vi "execute.vi"(8 "error in (no error)":errorcluster, 9 "trajectory in":refnum<class "GenericComponent.lvclass">, 10 "imaging mode in":refnum<class "GenericComponent.lvclass">, 11 "adapter in":refnum<class "AdapterTS090826ImagingModeToTrajectory.lvclass">) -> (0 "error out":errorcluster, 1 "trajectory out":refnum<class "GenericComponent.lvclass">, 2 "imaging mode out":refnum<class "GenericComponent.lvclass">, 3 "adapter out":refnum<class "AdapterTS090826ImagingModeToTrajectory.lvclass">)   [LabVIEW 2010, in "AdapterTS090826ImagingModeToTrajectory.lvclass"]
uses:
  AdapterTS090826ImagingModeToTrajectory.lvclass
  common/classes/GenericComponent/GenericComponent/GenericComponent.lvclass
  ImagingMode/ImagingModeTS090821Circular2D/ImagingModeTS090821Circular2D/ImagingModeTS090821Circular2D.lvclass
  Trajectory/TrajectoryTS090820Circular2D/TrajectoryTS090820Circular2D/TrajectoryTS090820Circular2D.lvclass
panel:
  # "imaging mode: ImagingModeTS090821Circular2D\ntrajectory: TrajectoryTS090820Circular2D"
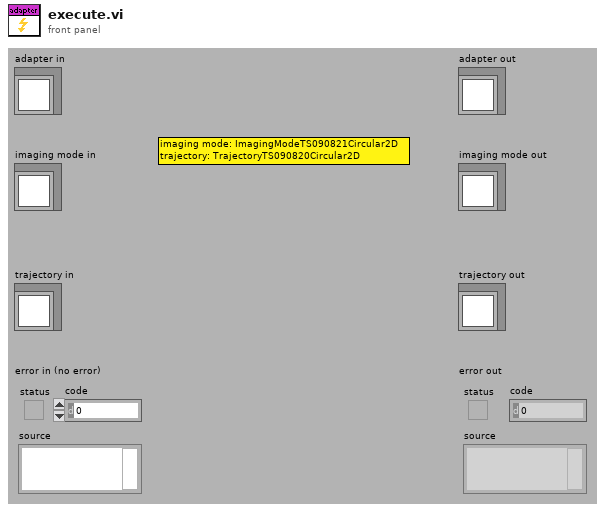
[diagram p1: front panel]
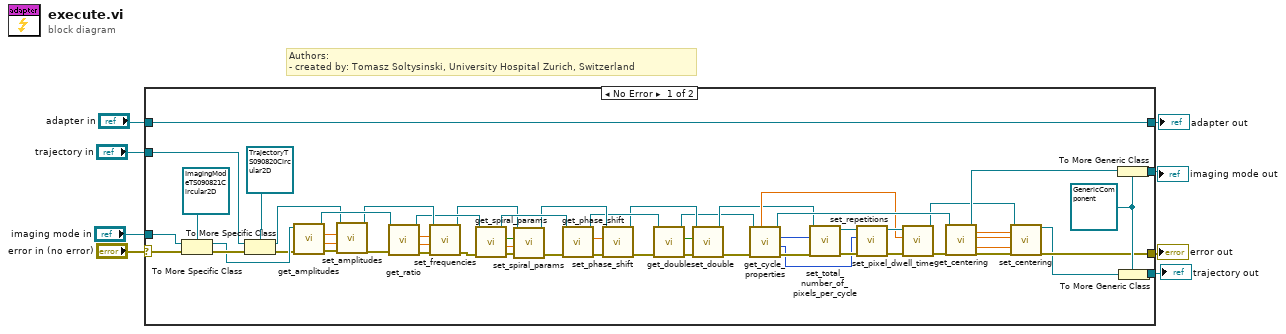
[diagram p0: block diagram]
diagram:
  # "Authors: \n- created by: Tomasz Soltysinski, University Hospital Zurich, Switzerland"
  n1 = case shown="No Error" "error in (no error)" {
    selector: "error in (no error)" -> [w65 w70]
    tunnel: [w67 w71] -> w6
    tunnel: "adapter in" -> [w67 w71]
    tunnel: "imaging mode in" -> [w66 w68]
    tunnel: "trajectory in" -> [w63 w69]
    tunnel: [w53 w68] -> w2
    tunnel: [w33 w70] -> w3
    tunnel: [w54 w69] -> w1
    frame No Error {
      w60 = refnum<class "GenericComponent.lvclass"> refnum ("GenericComponent.lvclass")
      n2 = To More Specific Class(target class=refnum<class "ImagingModeTS090821Circular2D.lvclass"> refnum, reference=w66, error in=w65) -> (specific class reference=w59:refnum<class "ImagingModeTS090821Circular2D.lvclass">, error out=w64:errorcluster)
      n3 = To More Specific Class(target class=refnum<class "TrajectoryTS090820Circular2D.lvclass"> refnum, reference=w63, error in=w64) -> (specific class reference=w42:refnum<class "TrajectoryTS090820Circular2D.lvclass">, error out=w57:errorcluster)
      n4 = call-dynamic "get_amplitudes.vi"("error in (no error)"=w57, "ScanModeTS090821Circular2D in"=w59) -> ("error out"=w49:errorcluster, "y amplitude"=w45:dbl[unit], "x amplitude"=w46:dbl[unit], "ScanModeTS090821Circular2D out"=w58:refnum<class "ImagingModeTS090821Circular2D.lvclass">)  [unwired: 6 in]
      n5 = call-dynamic "set_amplitudes.vi"("error in (no error)"=w49, "y amplitude"=w45, "x amplitude"=w46, "TrajectoryTS090820Circular2D in"=w42) -> ("error out"=w48:errorcluster, "TrajectoryTS090820Circular2D out"=w50:refnum<class "TrajectoryTS090820Circular2D.lvclass">)  [unwired: 6 in]
      n6 = call-dynamic "get_ratio.vi"("error in (no error)"=w48, "ScanModeTS090821Circular2D in"=w58) -> ("error out"=w47:errorcluster, "y frequency"=w43:dbl, "x frequency"=w44:dbl, "ScanModeTS090821Circular2D out"=w19:refnum<class "ImagingModeTS090821Circular2D.lvclass">)  [unwired: 6 in]
      n7 = call-dynamic "set_frequencies.vi"("error in (no error)"=w47, "y frequency"=w43, "x frequency"=w44, "TrajectoryTS090820Circular2D in"=w50) -> ("error out"=w20:errorcluster, "TrajectoryTS090820Circular2D out"=w18:refnum<class "TrajectoryTS090820Circular2D.lvclass">)  [unwired: 6 in]
      n8 = call-dynamic "get_spiral_params.vi"("error in (no error)"=w20, "ScanModeTS090821Circular2D in"=w19) -> ("error out"=w24:errorcluster, "dump factor"=w21:dbl, "Spiral"=w22:bool, "ScanModeTS090821Circular2D out"=w26:refnum<class "ImagingModeTS090821Circular2D.lvclass">)  [unwired: 6 in]
      n9 = call-dynamic "set_spiral_params.vi"("error in (no error)"=w24, "dump factor"=w21, "Spiral"=w22, "TrajectoryTS090820Circular2D in"=w18) -> ("error out"=w23:errorcluster, "TrajectoryTS090820Circular2D out"=w25:refnum<class "TrajectoryTS090820Circular2D.lvclass">)  [unwired: 6 in]
      n10 = call-dynamic "get_phase_shift.vi"("error in (no error)"=w23, "ScanModeTS090821Circular2D in"=w26) -> ("error out"=w56:errorcluster, "phase shift"=w52:dbl, "ScanModeTS090821Circular2D out"=w16:refnum<class "ImagingModeTS090821Circular2D.lvclass">)  [unwired: 7 in]
      n11 = call-dynamic "set_phase_shift.vi"("error in (no error)"=w56, "Phase shift"=w52, "TrajectoryTS090820Circular2D in"=w25) -> ("error out"=w15:errorcluster, "TrajectoryTS090820Circular2D out"=w14:refnum<class "TrajectoryTS090820Circular2D.lvclass">)  [unwired: 7 in]
      n12 = call-dynamic "get_double.vi"("error in (no error)"=w15, "ImagingModeTS090821Circular2D in"=w16) -> ("error out"=w12:errorcluster, "Double"=w10:bool, "ImagingModeTS090821Circular2D out"=w9:refnum<class "ImagingModeTS090821Circular2D.lvclass">)  [unwired: 7 in]
      n13 = call-dynamic "set_double.vi"("error in (no error)"=w12, "double"=w10, "TrajectoryTS090820Circular2D in"=w14) -> ("error out"=w11:errorcluster, "TrajectoryTS090820Circular2D out"=w13:refnum<class "TrajectoryTS090820Circular2D.lvclass">)  [unwired: 7 in]
      n14 = call-dynamic "get_cycle_properties.vi"("error in (no error)"=w11, "ScanModeTS090821Circular2D in"=w9) -> ("error out"=w55:errorcluster, "number of cycles"=w37:i32, "total number of pixels per cycle"=w51:i32, "ScanModeTS090821Circular2D out"=w32:refnum<class "ImagingModeTS090821Circular2D.lvclass">, "pixel dwell time"=w17:dbl[unit])  [unwired: 3 in, 2 out]
      n15 = call-dynamic "set_total_number_of_pixels_per_cycle.vi"("error in (no error)"=w55, "total number of pixels per cycle"=w51, "TrajectoryTS090820Circular2D in"=w13) -> ("error out"=w41:errorcluster, "TrajectoryTS090820Circular2D out"=w40:refnum<class "TrajectoryTS090820Circular2D.lvclass">)  [unwired: 7 in]
      n16 = call-dynamic "set_repetitions.vi"("error in (no error)"=w41, "repetitions"=w37, "GenericTrajectory in"=w40) -> ("error out"=w38:errorcluster, "GenericTrajectory out"=w39:refnum<class "TrajectoryTS090820Circular2D.lvclass">)  [unwired: 7 in]
      n17 = call-dynamic "set_pixel_dwell_time.vi"("error in (no error)"=w38, "pixel dwell time"=w17, "GenericTrajectory.lvclass in"=w39) -> ("error out"=w36:errorcluster, "GenericTrajectory.lvclass out"=w31:refnum<class "TrajectoryTS090820Circular2D.lvclass">)  [unwired: 7 in]
      n18 = call-dynamic "get_centering.vi"("ScanModeTS090821Circular2D in"=w32, "error in (no error)"=w36) -> ("ScanModeTS090821Circular2D out"=w35:refnum<class "ImagingModeTS090821Circular2D.lvclass">, "x center"=w30:dbl, "y center"=w29:dbl, "rotation angle"=w28:dbl, "error out"=w34:errorcluster)  [unwired: 13 in]
      n19 = call-dynamic "set_centering.vi"("TrajectoryTS090820Circular2D in"=w31, "x center"=w30, "y center"=w29, "rotation angle"=w28, "error in (no error)"=w34) -> ("TrajectoryTS090820Circular2D out"=w27:refnum<class "TrajectoryTS090820Circular2D.lvclass">, "error out"=w33:errorcluster)  [unwired: 13 in]
      n20 = To More Generic Class(target class=w60, reference=w35) -> (generic class reference=w53:refnum<class "GenericComponent.lvclass">)
      n21 = To More Generic Class(target class=w60, reference=w27) -> (generic class reference=w54:refnum<class "GenericComponent.lvclass">)
    }
    frame Error {
    }
  }
  "error out" <- w3
  "adapter out" <- w6
  "imaging mode out" <- w2
  "trajectory out" <- w1
